vi "Simple GUI.vi"() -> ()   [LabVIEW 2016]
panel:
  in  "Display":string
  in  "=":bool
  in  "x²":bool
  in  "+":bool
  in  "-":bool
  in  "x":bool
  in  "÷":bool
  in  "C":bool
  in  ".":bool
  in  "0":bool
  in  "3":bool
  in  "2":bool
  in  "1":bool
  in  "6":bool
  in  "5":bool
  in  "4":bool
  in  "9":bool
  in  "8":bool
  in  "7":bool
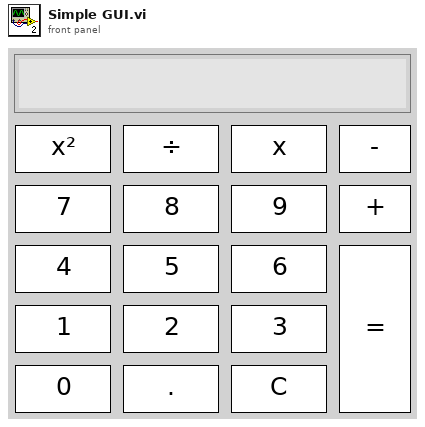
[diagram p1: front panel]
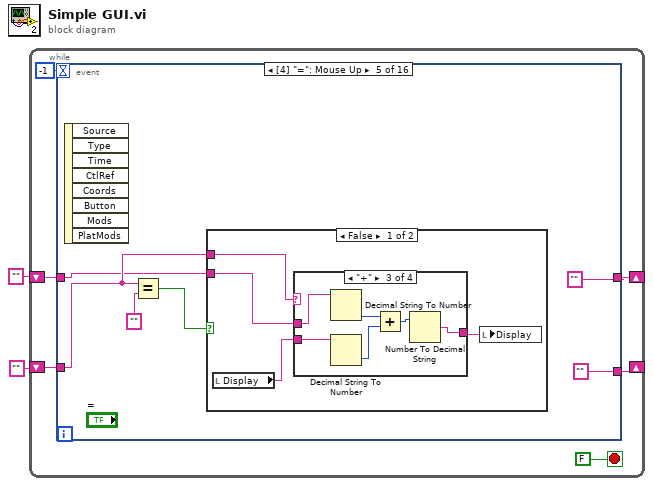
[diagram p0: block diagram]
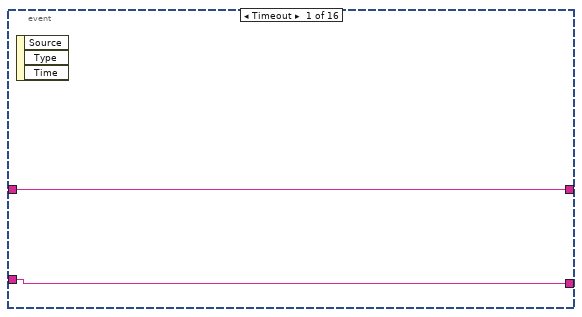
[diagram p2: hidden frame]
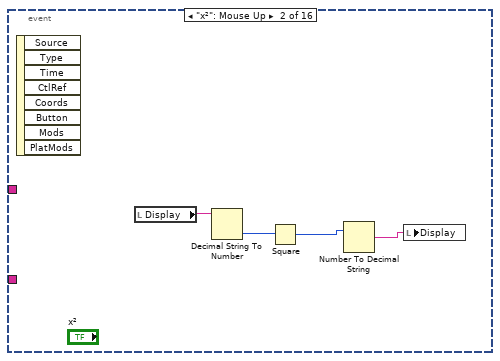
[diagram p3: hidden frame]
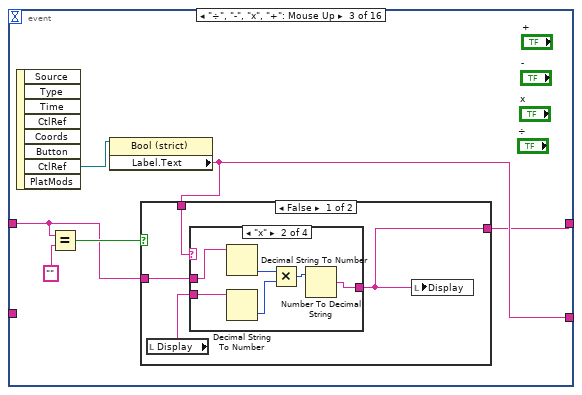
[diagram p4: hidden frame]
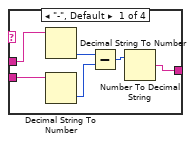
[diagram p5: hidden frame]
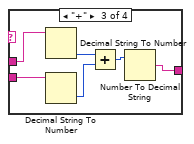
[diagram p6: hidden frame]
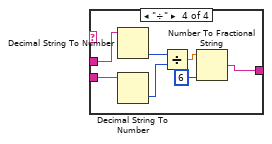
[diagram p7: hidden frame]
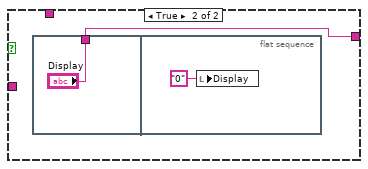
[diagram p8: hidden frame]
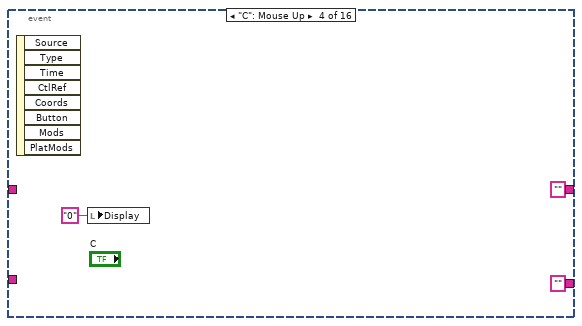
[diagram p9: hidden frame]
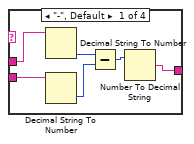
[diagram p10: hidden frame]
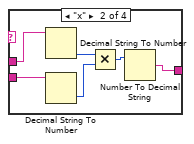
[diagram p11: hidden frame]
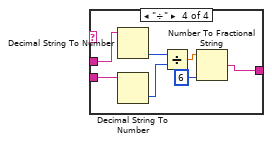
[diagram p12: hidden frame]
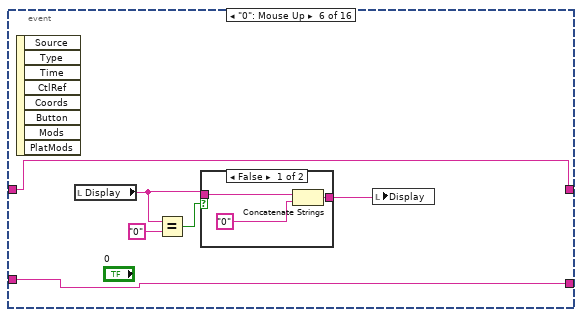
[diagram p14: hidden frame]
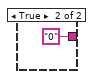
[diagram p15: hidden frame]
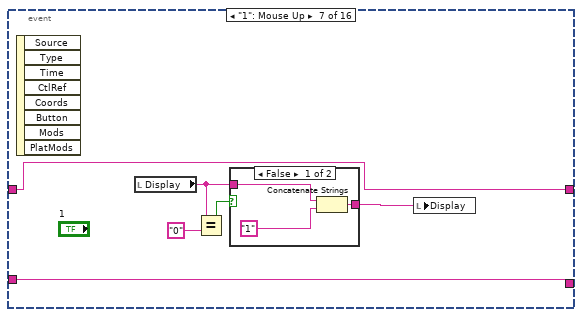
[diagram p16: hidden frame]
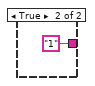
[diagram p17: hidden frame]
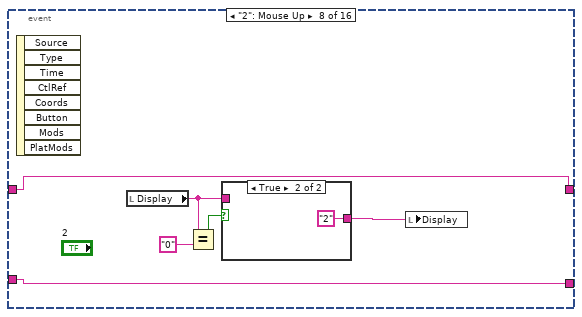
[diagram p18: hidden frame]
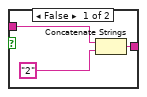
[diagram p19: hidden frame]
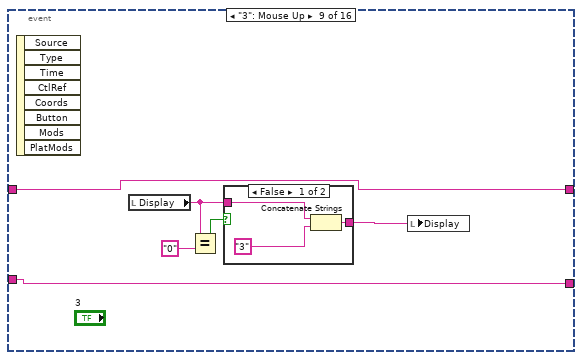
[diagram p20: hidden frame]
diagram:
  n1 = while {
    shift-right: [w3] -> _
    shift-left: "" ("Display") -> [w6]
    shift-right: [w4] -> _
    shift-left: "" ("Display") -> [w5]
    stop <- FALSE stop-if-true
    n2 = event shown="[4] \"=\": Mouse Up" {
      selector: _ -> [_ _ _ _ _ _ _ _ _ _ _ _ _ _ _ _]
      dyn-events: _ -> [_ _ _ _ _ _ _ _ _ _ _ _ _ _ _ _]
      timeout: -1 -> [_ _ _ _ _ _ _ _ _ _ _ _ _ _ _ _]
      tunnel: w6 -> [w10 _ w17 _ w57 w92 w102 w112 w122 w132 w142 w152 w162 w172 w182 w192]
      tunnel: w5 -> [w9 _ _ _ w58 w91 w101 w111 w121 w131 w141 w151 w161 w171 w181 w191]
      tunnel: [w9 _ w16 "" ("Label.Text") "" ("Label.Text") w91 w101 w111 w121 w131 w141 w151 w161 w171 w181 w191] -> w4
      tunnel: [w10 _ w15 "" ("Label.Text") "" ("Label.Text") w92 w102 w112 w122 w132 w142 w152 w162 w172 w182 w192] -> w3
      event Timeout {
        n3 = event-data() -> ()  [unwired: 1 in, 3 out]
      }
      event "x²": Mouse Up {
        n4 = event-data() -> ()  [unwired: 1 in, 8 out]
        n5 = local read "Display"() -> (w14:string)
        n6 = Decimal String To Number(string=w14) -> (number=w13:i32)  [unwired: 2 in, 1 out]
        n7 = Square(x=w13) -> (x^2=w12:i32)
        n8 = Number To Decimal String(number=w12) -> (decimal integer string=w11:string)  [unwired: 1 in]
        n9 = local write "Display"(w11) -> ()
      }
      event "÷", "-", "x", "+": Mouse Up {
        n10 = event-data() -> ("CtlRef"=w18:refnum<vi>)  [unwired: 1 in, 7 out]
        n11 = Equal?(x=w17, y="" ("Display")) -> (x = y?=w19:bool)
        n12 = property class="Bool (strict)"(reference=w18) -> ("Label.Text"=w16:string)  [unwired: 1 in, 2 out]
        n13 = case shown="False" w19 {
          tunnel: w16 -> [w24 _]
          tunnel: w17 -> [w23 _]
          tunnel: [w21 w50] -> w15
          frame False {
            n14 = local read "Display"() -> (w22:string)
            n15 = case shown="\"x\"" w24 {
              tunnel: w23 -> [w27 w33 w39 w49]
              tunnel: w22 -> [w26 w32 w38 w48]
              tunnel: [w25 w31 w37 w43] -> w21
              frame "-", Default {
                n16 = Decimal String To Number(string=w27) -> (number=w30:i32)  [unwired: 2 in, 1 out]
                n17 = Decimal String To Number(string=w26) -> (number=w29:i32)  [unwired: 2 in, 1 out]
                n18 = Subtract(x=w30, y=w29) -> (x-y=w28:i32)
                n19 = Number To Decimal String(number=w28) -> (decimal integer string=w25:string)  [unwired: 1 in]
              }
              frame "x" {
                n20 = Decimal String To Number(string=w33) -> (number=w36:i32)  [unwired: 2 in, 1 out]
                n21 = Decimal String To Number(string=w32) -> (number=w35:i32)  [unwired: 2 in, 1 out]
                n22 = Multiply(x=w36, y=w35) -> (x*y=w34:i32)
                n23 = Number To Decimal String(number=w34) -> (decimal integer string=w31:string)  [unwired: 1 in]
              }
              frame "+" {
                n24 = Decimal String To Number(string=w39) -> (number=w42:i32)  [unwired: 2 in, 1 out]
                n25 = Decimal String To Number(string=w38) -> (number=w41:i32)  [unwired: 2 in, 1 out]
                n26 = Add(x=w42, y=w41) -> (x+y=w40:i32)
                n27 = Number To Decimal String(number=w40) -> (decimal integer string=w37:string)  [unwired: 1 in]
              }
              frame "÷" {
                n28 = Decimal String To Number(string=w49) -> (number=w47:i32)  [unwired: 2 in, 1 out]
                n29 = Decimal String To Number(string=w48) -> (number=w46:i32)  [unwired: 2 in, 1 out]
                n30 = Divide(x=w47, y=w46) -> (x/y=w45:dbl)
                n31 = Number To Fractional String(number=w45, precision (6)=i16 6) -> (F-format string=w43:string)  [unwired: 2 in]
              }
            }
            n32 = local write "Display"(w21) -> ()
          }
          frame True {
            n33 = flat-sequence {
              tunnel: ["Display"] -> w50
              frame #0 {
              }
              frame #1 {
                n34 = local write "Display"("0" ("Display")) -> ()
              }
            }
          }
        }
      }
      event "C": Mouse Up {
        n35 = event-data() -> ()  [unwired: 1 in, 8 out]
        n36 = local write "Display"("0" ("Display")) -> ()
      }
      event "=": Mouse Up {
        n37 = event-data() -> ()  [unwired: 1 in, 8 out]
        n38 = Equal?(x=w58, y="" ("Display")) -> (x = y?=w60:bool)
        n39 = case shown="False" w60 {
          tunnel: w58 -> [w65 _]
          tunnel: w57 -> [w64 _]
          frame False {
            n40 = local read "Display"() -> (w63:string)
            n41 = case shown="\"+\"" w65 {
              tunnel: w64 -> [w68 w74 w80 w90]
              tunnel: w63 -> [w67 w73 w79 w89]
              tunnel: [w66 w72 w78 w84] -> w62
              frame "-", Default {
                n42 = Decimal String To Number(string=w68) -> (number=w71:i32)  [unwired: 2 in, 1 out]
                n43 = Decimal String To Number(string=w67) -> (number=w70:i32)  [unwired: 2 in, 1 out]
                n44 = Subtract(x=w71, y=w70) -> (x-y=w69:i32)
                n45 = Number To Decimal String(number=w69) -> (decimal integer string=w66:string)  [unwired: 1 in]
              }
              frame "x" {
                n46 = Decimal String To Number(string=w74) -> (number=w77:i32)  [unwired: 2 in, 1 out]
                n47 = Decimal String To Number(string=w73) -> (number=w76:i32)  [unwired: 2 in, 1 out]
                n48 = Multiply(x=w77, y=w76) -> (x*y=w75:i32)
                n49 = Number To Decimal String(number=w75) -> (decimal integer string=w72:string)  [unwired: 1 in]
              }
              frame "+" {
                n50 = Decimal String To Number(string=w80) -> (number=w83:i32)  [unwired: 2 in, 1 out]
                n51 = Decimal String To Number(string=w79) -> (number=w82:i32)  [unwired: 2 in, 1 out]
                n52 = Add(x=w83, y=w82) -> (x+y=w81:i32)
                n53 = Number To Decimal String(number=w81) -> (decimal integer string=w78:string)  [unwired: 1 in]
              }
              frame "÷" {
                n54 = Decimal String To Number(string=w90) -> (number=w88:i32)  [unwired: 2 in, 1 out]
                n55 = Decimal String To Number(string=w89) -> (number=w87:i32)  [unwired: 2 in, 1 out]
                n56 = Divide(x=w88, y=w87) -> (x/y=w86:dbl)
                n57 = Number To Fractional String(number=w86, precision (6)=i16 6) -> (F-format string=w84:string)  [unwired: 2 in]
              }
            }
            n58 = local write "Display"(w62) -> ()
          }
          frame True {
          }
        }
      }
      event "0": Mouse Up {
        n59 = event-data() -> ()  [unwired: 1 in, 8 out]
        n60 = local read "Display"() -> (w95:string)
        n61 = Equal?(x=w95, y="0") -> (x = y?=w93:bool)
        n62 = case shown="False" w93 {
          tunnel: w95 -> [w98 _]
          tunnel: [w97 "0"] -> w96
          frame False {
            n63 = Concatenate Strings(w98, "0") -> (w97:string)
          }
          frame True {
          }
        }
        n64 = local write "Display"(w96) -> ()
      }
      event "1": Mouse Up {
        n65 = event-data() -> ()  [unwired: 1 in, 8 out]
        n66 = local read "Display"() -> (w104:string)
        n67 = Equal?(x=w104, y="0") -> (x = y?=w103:bool)
        n68 = case shown="False" w103 {
          tunnel: [w108 "1"] -> w106
          tunnel: w104 -> [w107 _]
          frame False {
            n69 = Concatenate Strings(w107, "1") -> (w108:string)
          }
          frame True {
          }
        }
        n70 = local write "Display"(w106) -> ()
      }
      event "2": Mouse Up {
        n71 = event-data() -> ()  [unwired: 1 in, 8 out]
        n72 = local read "Display"() -> (w114:string)
        n73 = Equal?(x=w114, y="0") -> (x = y?=w113:bool)
        n74 = case shown="True" w113 {
          tunnel: [w118 "2"] -> w116
          tunnel: w114 -> [w117 _]
          frame False {
            n75 = Concatenate Strings(w117, "2") -> (w118:string)
          }
          frame True {
          }
        }
        n76 = local write "Display"(w116) -> ()
      }
      event "3": Mouse Up {
        n77 = event-data() -> ()  [unwired: 1 in, 8 out]
        n78 = local read "Display"() -> (w124:string)
        n79 = Equal?(x=w124, y="0") -> (x = y?=w123:bool)
        n80 = case shown="False" w123 {
          tunnel: [w128 "3"] -> w126
          tunnel: w124 -> [w127 _]
          frame False {
            n81 = Concatenate Strings(w127, "3") -> (w128:string)
          }
          frame True {
          }
        }
        n82 = local write "Display"(w126) -> ()
      }
      event "4": Mouse Up {
        n83 = event-data() -> ()  [unwired: 1 in, 8 out]
        n84 = local read "Display"() -> (w134:string)
        n85 = Equal?(x=w134, y="0") -> (x = y?=w133:bool)
        n86 = case shown="False" w133 {
          tunnel: [w138 "4"] -> w136
          tunnel: w134 -> [w137 _]
          frame False {
            n87 = Concatenate Strings(w137, "4") -> (w138:string)
          }
          frame True {
          }
        }
        n88 = local write "Display"(w136) -> ()
      }
      event "5": Mouse Up {
        n89 = event-data() -> ()  [unwired: 1 in, 8 out]
        n90 = local read "Display"() -> (w144:string)
        n91 = Equal?(x=w144, y="0") -> (x = y?=w143:bool)
        n92 = case shown="False" w143 {
          tunnel: [w148 "5"] -> w146
          tunnel: w144 -> [w147 _]
          frame False {
            n93 = Concatenate Strings(w147, "5") -> (w148:string)
          }
          frame True {
          }
        }
        n94 = local write "Display"(w146) -> ()
      }
      event "6": Mouse Up {
        n95 = event-data() -> ()  [unwired: 1 in, 8 out]
        n96 = local read "Display"() -> (w154:string)
        n97 = Equal?(x=w154, y="0") -> (x = y?=w153:bool)
        n98 = case shown="False" w153 {
          tunnel: [w158 "6"] -> w156
          tunnel: w154 -> [w157 _]
          frame False {
            n99 = Concatenate Strings(w157, "6") -> (w158:string)
          }
          frame True {
          }
        }
        n100 = local write "Display"(w156) -> ()
      }
      event "7": Mouse Up {
        n101 = event-data() -> ()  [unwired: 1 in, 8 out]
        n102 = local read "Display"() -> (w164:string)
        n103 = Equal?(x=w164, y="0") -> (x = y?=w163:bool)
        n104 = case shown="False" w163 {
          tunnel: [w168 "7"] -> w166
          tunnel: w164 -> [w167 _]
          frame False {
            n105 = Concatenate Strings(w167, "7") -> (w168:string)
          }
          frame True {
          }
        }
        n106 = local write "Display"(w166) -> ()
      }
      event "8": Mouse Up {
        n107 = event-data() -> ()  [unwired: 1 in, 8 out]
        n108 = local read "Display"() -> (w174:string)
        n109 = Equal?(x=w174, y="0") -> (x = y?=w173:bool)
        n110 = case shown="False" w173 {
          tunnel: [w178 "8"] -> w176
          tunnel: w174 -> [w177 _]
          frame False {
            n111 = Concatenate Strings(w177, "8") -> (w178:string)
          }
          frame True {
          }
        }
        n112 = local write "Display"(w176) -> ()
      }
      event "9": Mouse Up {
        n113 = event-data() -> ()  [unwired: 1 in, 8 out]
        n114 = local read "Display"() -> (w184:string)
        n115 = Equal?(x=w184, y="0") -> (x = y?=w183:bool)
        n116 = case shown="False" w183 {
          tunnel: [w188 "9"] -> w186
          tunnel: w184 -> [w187 _]
          frame False {
            n117 = Concatenate Strings(w187, "9") -> (w188:string)
          }
          frame True {
          }
        }
        n118 = local write "Display"(w186) -> ()
      }
      event ".": Mouse Up {
        n119 = event-data() -> ()  [unwired: 1 in, 8 out]
      }
    }
  }
